vi "TCPIPCommunication.vi"() -> ()   [LabVIEW 2024]
uses:
  TCPIP Actor/TCP Multiple Connections Data.ctl
  Control/TCPIP CMD.ctl
  PCAN/CAN Communication.llb/@Parameter_MTEST.vi
panel:
  in  "Clients":i32(listbox)
  out "error out":errorcluster
  out "ServerIsListening":bool
  in  "port":u16=8082
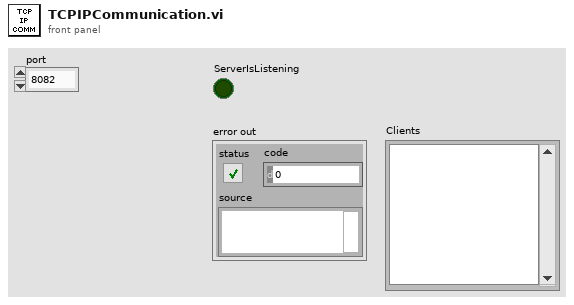
[diagram p1: front panel]
types:
  T1 = typedef "TCPIP CMD.ctl" = enum16{"None", "REMOTE", "LOCAL", "ERES", "ERROR?", "SERVO", "SERVO?", "DIRN", "DIRN?", "TESTMODE", "TESTMODE?", "SPEED", "SPEED?", "TORQUE", "TORQUE?", "POSITION", "POSRES", "TPS", "TPS?", "PS", "PS?", "PSON", "PSOFF", "COLUMNS", "DATA", "RAMP", "STOP", "DISCONN", "STARTLOG", "STOPLOG"}
  T2 = typedef "TCP Multiple Connections Data.ctl" = cluster{"Clients":refnum<k5>[], "Listener":refnum<k5>}
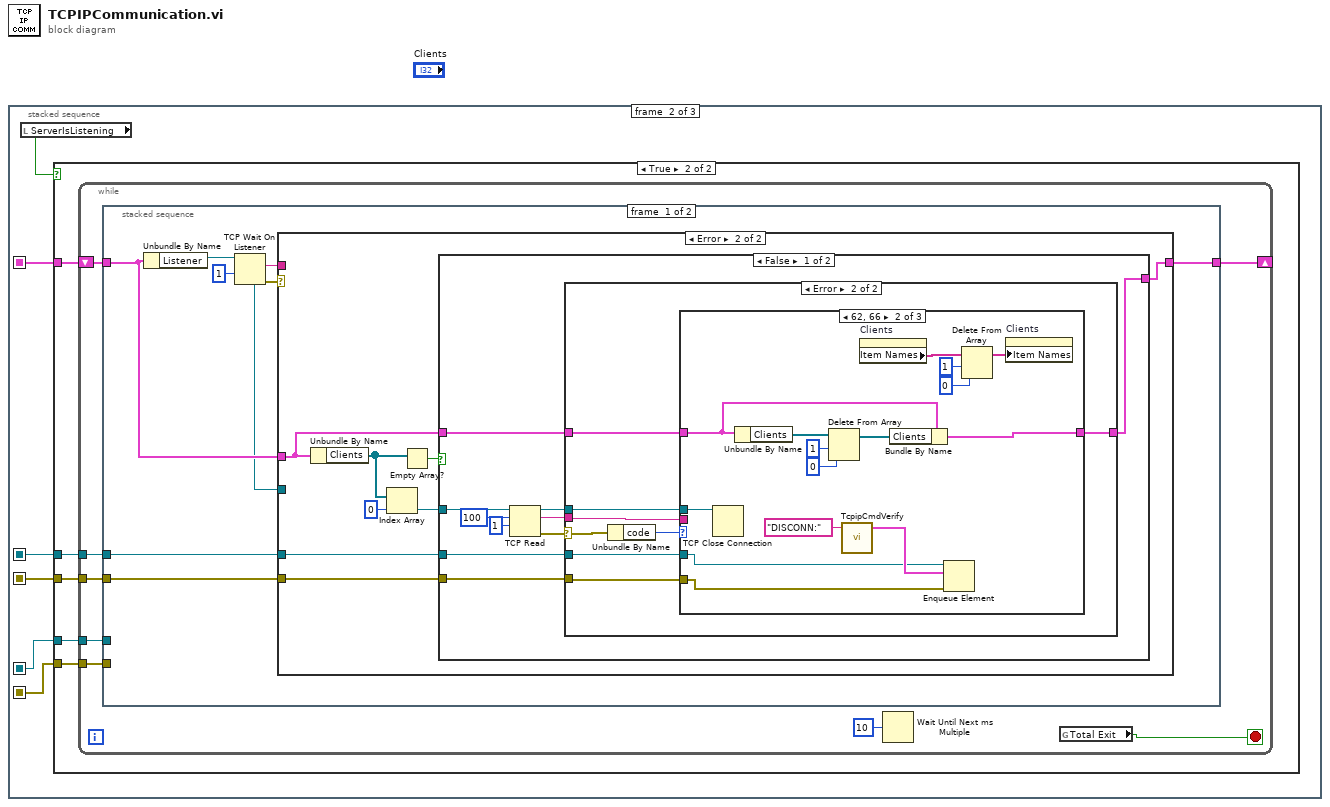
[diagram p0: block diagram]
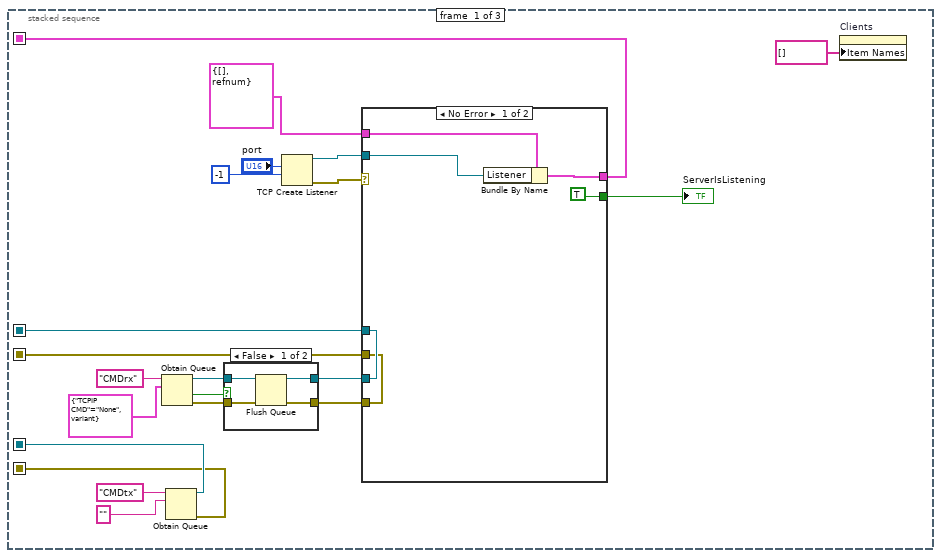
[diagram p2: hidden frame]
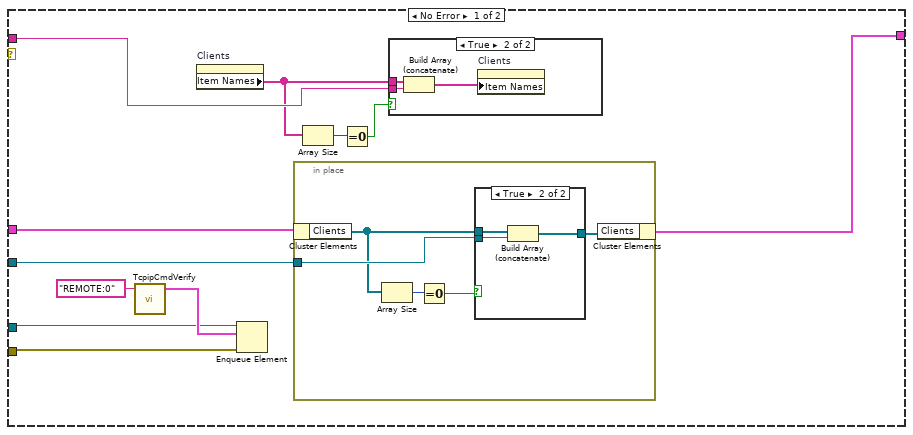
[diagram p6: hidden frame]
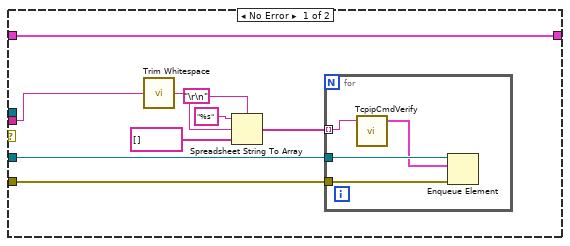
[diagram p9: hidden frame]
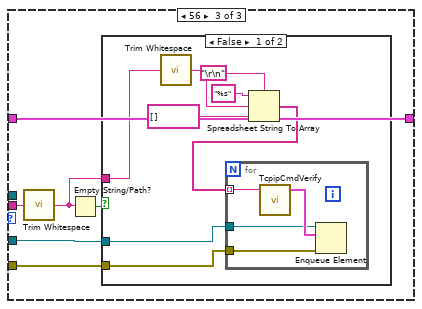
[diagram p11: hidden frame]
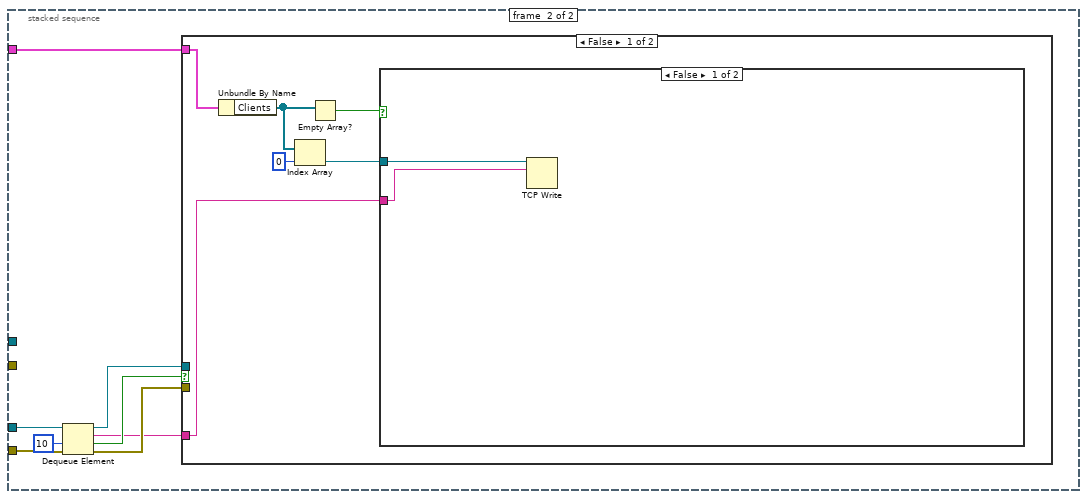
[diagram p14: hidden frame]
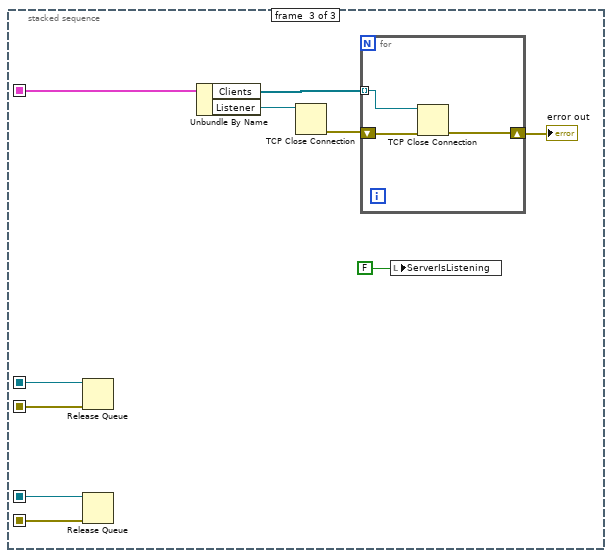
[diagram p17: hidden frame]
diagram:
  n1 = stacked-sequence {
    seq-local: [w15 _ _] -> [_ w41 w187]
    seq-local: [w7 _ _] -> [_ w40 w181]
    seq-local: [w6 _ _] -> [_ w39 w180]
    seq-local: [w9 _ _] -> [_ w38 w179]
    seq-local: [w8 _ _] -> [_ w37 w178]
    frame #0 {
      n2 = Obtain Queue(name (unnamed)="CMDrx", element data type=cluster{"TCPIP CMD":T1, variant} {"TCPIP CMD"=enum."None", variant}) -> (queue out=w4:refnum<queue>, created new?=w5:bool, error out=w3:errorcluster)  [unwired: 3 in]
      n3 = Obtain Queue(name (unnamed)="CMDtx", element data type="") -> (queue out=w9:refnum<queue>, error out=w8:errorcluster)  [unwired: 3 in, 1 out]
      n4 = case shown="False" w5 {
        tunnel: w4 -> [w23 w27]
        tunnel: w3 -> [w22 w26]
        tunnel: [w24 w27] -> w2
        tunnel: [w25 w26] -> w1
        frame False {
          n5 = Flush Queue(queue=w23, error in (no error)=w22) -> (queue out=w24:refnum<queue>, error out=w25:errorcluster)  [unwired: 1 out]
        }
        frame True {
        }
      }
      n6 = TCP Create Listener(9:-1 ("timeout ms (25000)"), 10:"port") -> (0:w19:errorcluster, 3:w17:refnum<k5>)  [unwired: 3 in, 1 out]
      n7 = case shown="No Error" w19 {
        tunnel: [TRUE _] -> w18
        tunnel: w17 -> [w31 _]
        tunnel: T2 {"Clients"=[], "Listener"=refnum} ("Data") -> [w32 w36]
        tunnel: [w30 w36] -> w15
        tunnel: w2 -> [w29 w35]
        tunnel: w1 -> [w28 w34]
        tunnel: [w29 w35] -> w7
        tunnel: [w28 w34] -> w6
        frame No Error {
          n8 = Bundle By Name(cluster=w32, "Listener"=w31) -> (w30:T2)
        }
        frame Error {
        }
      }
      "ServerIsListening" <- w18
      n9 = property on="Clients" class="LstBox (strict)"("Item Names"=string[] []) -> ()  [unwired: 2 in, 2 out]
    }
    frame #1 {
      n10 = local read "ServerIsListening"() -> (w42:bool)
      n11 = case shown="True" w42 {
        tunnel: w41 -> [_ w47]
        tunnel: w40 -> [_ w46]
        tunnel: w39 -> [_ w45]
        tunnel: w38 -> [_ w44]
        tunnel: w37 -> [_ w43]
        frame False {
        }
        frame True {
          n12 = while {
            shift-right: [w54] -> _
            shift-left: w47 -> [w55]
            tunnel: w46 -> [w53]
            tunnel: w45 -> [w52]
            tunnel: w44 -> [w51]
            tunnel: w43 -> [w50]
            stop <- w49 stop-if-true
            n13 = stacked-sequence {
              tunnel: w55 -> [w60 w162]
              tunnel: [w58 _] -> w54
              tunnel: w53 -> [w57 _]
              tunnel: w52 -> [w56 _]
              tunnel: w51 -> [_ w169]
              tunnel: w50 -> [_ w168]
              frame #0 {
                n14 = Unbundle By Name(w60) -> ("Listener"=w64:refnum<k5>)
                n15 = TCP Wait On Listener(9:1 ("timeout ms (wait forever: -1)"), 11:w64) -> (0:w62:errorcluster, 2:w61:string, 4:w59:refnum<k5>)  [unwired: 2 in, 2 out]
                n16 = case shown="Error" w62 {
                  tunnel: w61 -> [w72 _]
                  tunnel: w60 -> [w75 w94]
                  tunnel: w59 -> [w74 _]
                  tunnel: [w73 w93] -> w58
                  tunnel: w57 -> [w69 w89]
                  tunnel: w56 -> [w68 w88]
                  frame No Error {
                    n17 = call "TcpipCmdVerify.vi"("CMDrx"="REMOTE:0") -> ("QueneElement"=w71:cluster{"TCPIP CMD":T1, variant})  [unwired: 4 in]
                    n18 = property on="Clients" class="LstBox (strict)"() -> ("Item Names"=w67:string[])  [unwired: 2 in, 2 out]
                    n19 = Enqueue Element(queue=w69, element=w71, error in (no error)=w68) -> ()  [unwired: 1 in, 3 out]
                    n20 = in-place {
                      in-place-border: w74 -> [w82]
                      n21 = in-place-cluster #1(w75) -> ("Clients"=w81:refnum<k5>[])
                      n22 = Array Size(array=w81) -> (size(s)=w80:i32)
                      n23 = Equal To 0?(x=w80) -> (x = 0?=w79:bool)
                      n24 = case shown="True" w79 {
                        tunnel: [w84 w87] -> w83
                        tunnel: w82 -> [_ w86]
                        tunnel: w81 -> [w84 w85]
                        frame False {
                        }
                        frame True {
                          n25 = Build Array (concatenate)(w85, w86) -> (w87:refnum<k5>[])
                        }
                      }
                      n26 = in-place-cluster #1("Clients"=w83) -> (w73:T2)
                    }
                    n27 = Array Size(array=w67) -> (size(s)=w66:i32)
                    n28 = Equal To 0?(x=w66) -> (x = 0?=w65:bool)
                    n29 = case shown="True" w65 {
                      tunnel: w72 -> [_ w78]
                      tunnel: w67 -> [_ w76]
                      frame False {
                      }
                      frame True {
                        n30 = Build Array (concatenate)(w76, w78) -> (w77:string[])
                        n31 = property on="Clients" class="LstBox (strict)"("Item Names"=w77) -> ()  [unwired: 2 in, 2 out]
                      }
                    }
                  }
                  frame Error {
                    n32 = Unbundle By Name(w94) -> ("Clients"=w92:refnum<k5>[])
                    n33 = Index Array(array=w92, index=0) -> (element=w90:refnum<k5>)
                    n34 = Empty Array?(array=w92) -> (empty?=w95:bool)
                    n35 = case shown="False" w95 {
                      tunnel: [w98 w161] -> w93
                      tunnel: w94 -> [w99 w161]
                      tunnel: w90 -> [w105 _]
                      tunnel: w89 -> [w97 _]
                      tunnel: w88 -> [w96 _]
                      frame False {
                        n36 = TCP Read(connection ID=w105, bytes to read=100, 9:1 ("timeout ms (25000)")) -> (connection ID out=w101:refnum<k5>, data out=w100:string, error out=w102:errorcluster)  [unwired: 2 in]
                        n37 = case shown="Error" w102 {
                          selector: w102 -> [_ w126]
                          tunnel: w101 -> [_ w124]
                          tunnel: w100 -> [w107 w121]
                          tunnel: w99 -> [w114 w123]
                          tunnel: [w114 w122] -> w98
                          tunnel: w97 -> [w113 w120]
                          tunnel: w96 -> [w112 w119]
                          frame No Error {
                            n38 = call <vilib>:"Trim Whitespace.vi"("string"=w107) -> ("trimmed string"=w108:string)  [unwired: 1 in]
                            n39 = Spreadsheet String To Array(delimiter (Tab)="\r\n", format string="%s", spreadsheet string=w108, array type (2D Dbl)=string[] []) -> (array=w106:string[])
                            n40 = for {
                              tunnel: w113 -> [w118]
                              tunnel: w112 -> [w117]
                              tunnel: w106 -> [w115] mode=indexing
                              n41 = call "TcpipCmdVerify.vi"("CMDrx"=w115) -> ("QueneElement"=w116:cluster{"TCPIP CMD":T1, variant})  [unwired: 4 in]
                              n42 = Enqueue Element(queue=w118, element=w116, error in (no error)=w117) -> ()  [unwired: 1 in, 3 out]
                            }
                          }
                          frame Error {
                            n43 = Unbundle By Name(w126) -> ("code"=w125:i32)
                            n44 = case shown="62, 66" w125 {
                              tunnel: w124 -> [_ w142 _]
                              tunnel: w123 -> [w127 w138 w146]
                              tunnel: [w127 w136 w146] -> w122
                              tunnel: w121 -> [_ _ w145]
                              tunnel: w120 -> [_ w130 w148]
                              tunnel: w119 -> [_ w129 w147]
                              frame 0, Default {
                              }
                              frame 62, 66 {
                                n45 = TCP Close Connection(connection ID=w142) -> ()  [unwired: 2 in, 2 out]
                                n46 = Unbundle By Name(w138) -> ("Clients"=w141:refnum<k5>[])
                                n47 = Delete From Array(array=w141, length=1, index=0) -> (array with subset deleted=w137:refnum<k5>[])  [unwired: 1 out]
                                n48 = call "TcpipCmdVerify.vi"("CMDrx"="DISCONN:") -> ("QueneElement"=w131:cluster{"TCPIP CMD":T1, variant})  [unwired: 4 in]
                                n49 = property on="Clients" class="LstBox (strict)"() -> ("Item Names"=w135:string[])  [unwired: 2 in, 2 out]
                                n50 = Bundle By Name(cluster=w138, "Clients"=w137) -> (w136:T2)
                                n51 = Enqueue Element(queue=w130, element=w131, error in (no error)=w129) -> ()  [unwired: 1 in, 3 out]
                                n52 = Delete From Array(array=w135, length=1, index=0) -> (array with subset deleted=w132:string[])  [unwired: 1 out]
                                n53 = property on="Clients" class="LstBox (strict)"("Item Names"=w132) -> ()  [unwired: 2 in, 2 out]
                              }
                              frame 56 {
                                n54 = call <vilib>:"Trim Whitespace.vi"("string"=w145) -> ("trimmed string"=w143:string)  [unwired: 1 in]
                                n55 = Empty String/Path?(string/path=w143) -> (empty?=w144:bool)
                                n56 = case shown="False" w144 {
                                tunnel: w148 -> [w156 _]
                                tunnel: w147 -> [w155 _]
                                tunnel: w143 -> [w150 _]
                                frame False {
                                n57 = call <vilib>:"Trim Whitespace.vi"("string"=w150) -> ("trimmed string"=w151:string)  [unwired: 1 in]
                                n58 = Spreadsheet String To Array(delimiter (Tab)="\r\n", format string="%s", spreadsheet string=w151, array type (2D Dbl)=string[] []) -> (array=w149:string[])
                                n59 = for {
                                tunnel: w156 -> [w159]
                                tunnel: w155 -> [w158]
                                tunnel: w149 -> [w157] mode=indexing
                                n60 = call "TcpipCmdVerify.vi"("CMDrx"=w157) -> ("QueneElement"=w160:cluster{"TCPIP CMD":T1, variant})  [unwired: 4 in]
                                n61 = Enqueue Element(queue=w159, element=w160, error in (no error)=w158) -> ()  [unwired: 1 in, 3 out]
                                }
                                }
                                frame True {
                                }
                                }
                              }
                            }
                          }
                        }
                      }
                      frame True {
                      }
                    }
                  }
                }
              }
              frame #1 {
                n62 = Dequeue Element(queue=w169, timeout in ms (-1)=10, error in (no error)=w168) -> (queue out=w166:refnum<queue>, element=w163:string, timed out?=w165:bool, error out=w164:errorcluster)
                n63 = case shown="False" w165 {
                  tunnel: w166 -> [_ _]
                  tunnel: w164 -> [_ _]
                  tunnel: w163 -> [w170 _]
                  tunnel: w162 -> [w173 _]
                  frame False {
                    n64 = Unbundle By Name(w173) -> ("Clients"=w175:refnum<k5>[])
                    n65 = Index Array(array=w175, index=0) -> (element=w171:refnum<k5>)
                    n66 = Empty Array?(array=w175) -> (empty?=w172:bool)
                    n67 = case shown="False" w172 {
                      tunnel: w171 -> [w177 _]
                      tunnel: w170 -> [w176 _]
                      frame False {
                        n68 = TCP Write(connection ID=w177, data in=w176) -> ()  [unwired: 2 in, 3 out]
                      }
                      frame True {
                      }
                    }
                  }
                  frame True {
                  }
                }
              }
            }
            n69 = Wait Until Next ms Multiple(millisecond multiple=u32 10) -> ()  [unwired: 1 out]
            n70 = global read "@Parameter_MTEST.vi" "Total Exit"() -> (w49:bool)
          }
        }
      }
    }
    frame #2 {
      n71 = Release Queue(queue=w181, error in (no error)=w180) -> ()  [unwired: 1 in, 3 out]
      n72 = Release Queue(queue=w179, error in (no error)=w178) -> ()  [unwired: 1 in, 3 out]
      n73 = Unbundle By Name(w187) -> ("Clients"=w186:refnum<k5>[], "Listener"=w185:refnum<k5>)
      n74 = TCP Close Connection(connection ID=w185) -> (error out=w184:errorcluster)  [unwired: 2 in, 1 out]
      n75 = for {
        tunnel: w186 -> [w190] mode=indexing
        shift-right: [w188] -> w183
        shift-left: w184 -> [w189]
        n76 = TCP Close Connection(connection ID=w190, error in (no error)=w189) -> (error out=w188:errorcluster)  [unwired: 1 in, 1 out]
      }
      "error out" <- w183
      n77 = local write "ServerIsListening"(FALSE) -> ()
    }
  }
